vi "GlobalVariableTest.vi"() -> ()   [LabVIEW 2019]
panel:
  in  "Global_Variable":string
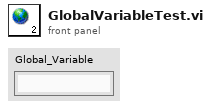
[diagram p1: front panel]
diagram:
